vi "IMAQ Write Image File(Float32 Ex) With Vision Info.vi"(8 "error in (no error)":errorcluster, 9 "Image Quality":u32=750 max=1000 step=10, 10 "File Path":path, 11 "Image":T1) -> (0 "error out":errorcluster, 3 "Image Out (duplicate)":T1)   [LabVIEW 2020]
uses:
  <vilib>/vision/Image Controls.llb/IMAQ Image.ctl
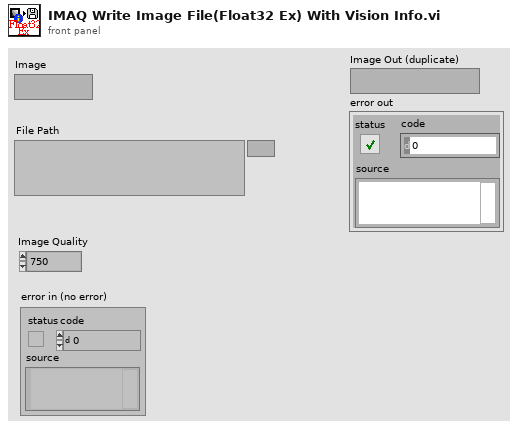
[diagram p1: front panel]
types:
  T1 = typedef "IMAQ Image.ctl" = refnum<image>
  T2 = typedef "Image Type" = u32
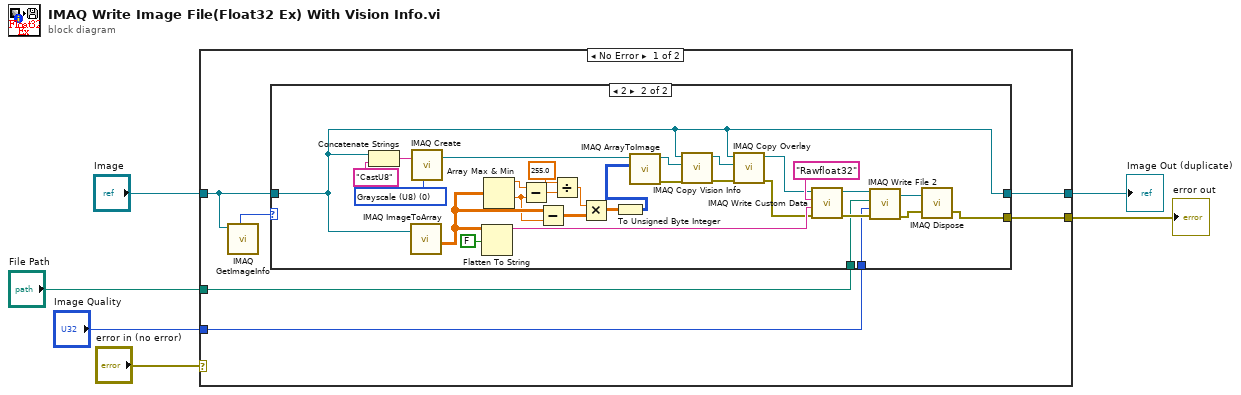
[diagram p0: block diagram]
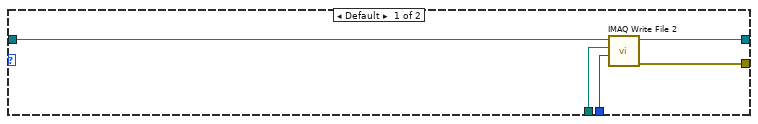
[diagram p2: hidden frame]
diagram:
  n1 = case shown="No Error" "error in (no error)" {
    selector: "error in (no error)" -> [_ w49]
    tunnel: "File Path" -> [w11 _]
    tunnel: [w10 w48] -> w5
    tunnel: [w9 w49] -> w4
    tunnel: "Image" -> [w8 w48]
    tunnel: "Image Quality" -> [w7 _]
    frame No Error {
      n2 = call "IMAQ GetImageInfo"("Image"=w8) -> ("Image Type"=w12:T2)  [unwired: 3 in, 7 out]
      n3 = case shown="2" w12 {
        tunnel: w8 -> [w17 w23]
        tunnel: w11 -> [w16 w40]
        tunnel: [w15 w23] -> w10
        tunnel: [w14 w27] -> w9
        tunnel: w7 -> [w13 w26]
        frame Default {
          n4 = call-poly "IMAQ Write File 2"("Image Quality"=w13, "File Path"=w16, "Image"=w17) -> ("error out"=w14:errorcluster, "Image Out (duplicate)"=w15:T1)  [unwired: 7 in]
        }
        frame 2 {
          w32 = T2 0 items=["Grayscale (U8)", "Grayscale (I16)", "Grayscale (SGL)", "Complex (CSG)", "RGB (U32)", "HSL (U32)", "RGB (U64)", "Grayscale (U16)"] ("Image Type")
          n5 = Concatenate Strings(w23, "CastU8" ("string")) -> (w34:string)
          n6 = call "IMAQ ImageToArray"("Image"=w23) -> ("Image Pixels (Float)"=w38:sgl[][])  [unwired: 3 in, 4 out]
          n7 = call "IMAQ Create"("Image Name"=w34, "Image Type"=w32) -> ("New Image"=w31:T1)  [unwired: 3 in, 1 out]
          n8 = Flatten To String(anything=w38, prepend array or string size? (T)=FALSE) -> (data string=w42:string)  [unwired: 2 in, 2 out]
          n9 = Array Max & Min(array=w38) -> (max value=w44:sgl, min value=w37:sgl)  [unwired: 2 out]
          n10 = Subtract(x=w44, y=w37) -> (x-y=w47:sgl)
          n11 = Subtract(x=w38, y=w37) -> (x-y=w36:sgl[][])
          n12 = Divide(x=sgl 255.0, y=w47) -> (x/y=w35:sgl)
          n13 = Multiply(x=w35, y=w36) -> (x*y=w30:sgl[][])
          n14 = To Unsigned Byte Integer(number=w30) -> (unsigned 8bit integer=w29:u8[][])
          n15 = call "IMAQ ArrayToImage"("Image Pixels (U8)"=w29, "Image"=w31) -> ("error out"=w20:errorcluster, "Image Out"=w25:T1)  [unwired: 8 in]
          n16 = call "IMAQ Copy Vision Info"("error in (no error)"=w20, "Image Dst"=w25, "Image Src"=w23) -> ("error out"=w24:errorcluster, "Image Dst Out"=w22:T1)  [unwired: 6 in, 1 out]
          n17 = call "IMAQ Copy Overlay"("error in (no error)"=w24, "Image Dst"=w22, "Image Src"=w23) -> ("error out"=w19:errorcluster, "Image Dst Out"=w21:T1)  [unwired: 7 in]
          n18 = call "IMAQ Write Custom Data"("error in (no error)"=w19, "Custom Data In"=w42, "Key"="Rawfloat32", "Image"=w21) -> ("error out"=w41:errorcluster, "Image Out"=w39:T1)  [unwired: 6 in]
          n19 = call-poly "IMAQ Write File 2"("error in (no error)"=w41, "Image Quality"=w26, "File Path"=w40, "Image"=w39) -> ("error out"=w28:errorcluster, "Image Out (duplicate)"=w18:T1)  [unwired: 6 in]
          n20 = call "IMAQ Dispose"("Image"=w18, "error in (no error)"=w28) -> ("error out"=w27:errorcluster)  [unwired: 4 in]
        }
      }
    }
    frame Error {
    }
  }
  "Image Out (duplicate)" <- w5
  "error out" <- w4
